vi "Generate GIS Script.vi"(7 "TopLevel in":refnum<class "TopLevel.lvclass">, 8 "error in":errorcluster, 11 "Priming API Data":T1={"Interval (s)"=0.0, "PurgeDuration (s)"=0.0, "Repeats"=0, "PrimingMode"=enum."Pre-Purge", "Head"=enum."1", "Frequency (Hz)"=0, "PrintWeight"=0.1}) -> (0 "error out":errorcluster, 2 "GIS Script":string[](array[string]), 3 "PPScanTrk":T4, 5 "TopLevel out":refnum<class "TopLevel.lvclass">)   [LabVIEW 2022 SP3, in "TopLevel.lvclass"]
uses:
  TopLevel.lvclass
  Typedefs/PrepurgeScanTracking--Cluster.ctl
  Typedefs/PrimingMode APIData.ctl
  Typedefs/PurgeMode--Enum.ctl
  Typedefs/PrinterHeads--Enum.ctl
  IO/Typedefs/ICP1-D0 Channel Names.ctl
  IO/IO.lvclass
panel:
  out "number of replacements":i32
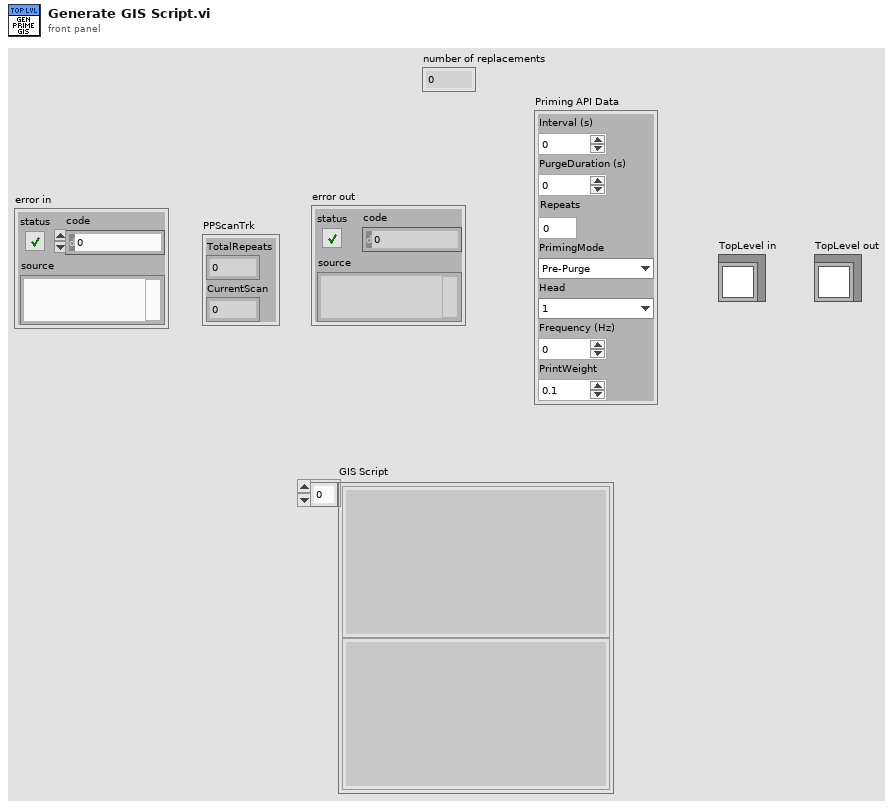
[diagram p1: front panel]
types:
  T1 = typedef "TopLevel.lvclass/PrimingMode APIData.ctl" = cluster{"Interval (s)":dbl, "PurgeDuration (s)":dbl, "Repeats":u8, "PrimingMode":T2, "Head":T3, "Frequency (Hz)":i32, "PrintWeight":dbl}
  T2 = typedef "PurgeMode--Enum.ctl" = enum16{"Pre-Purge", "Purge", "Spit", "Shake"}
  T3 = typedef "PrinterHeads--Enum.ctl" = enum16{"-1", "1", "2", "3", "4", "5", "6"}
  T4 = typedef "PrepurgeScanTracking--Cluster.ctl" = cluster{"TotalRepeats":i32, "CurrentScan":i32}
  T5 = typedef "IO.lvclass/ICP1-D0 Channel Names.ctl" = enum16{"None", "Meniscus Pressure Reg PWR - R1", "Meniscus Pressure Reg PWR - R2", "Meniscus Pressure Reg PWR - R3", "Meniscus Pressure Reg PWR - R4", "Meniscus Pressure Reg PWR - R5", "Meniscus Pressure Reg PWR - R6", "Clear Stage Alarm", "Servo ON", "Purge Valve Open - R1", "Purge Valve Open - R2", "Purge Valve Open - R3", "Purge Valve Open - R4", "Purge Valve Open - R5", "Purge Valve Open - R6"}
  T6 = typedef "DLPConfig)Init_HeadPropertyAttr--Cluster.ctl" = cluster{"HeadNumber":u8, "Material":string, "HeadLocalX":dbl, "HeadLocalY":dbl, "HeadRotationAngle":dbl, "VH2L_Hi":dbl, "VH2R_Hi":dbl, "VH1LA_Hi":dbl, "VH1LB_Hi":dbl, "VH1RA_Hi":dbl, "VH1RB_Hi":dbl, "VH2L_Lo":dbl, "VH2R_Lo":dbl, "VH1LA_Lo":dbl, "VH1LB_Lo":dbl, "VH1RA_Lo":dbl, "VH1RB_Lo":dbl}
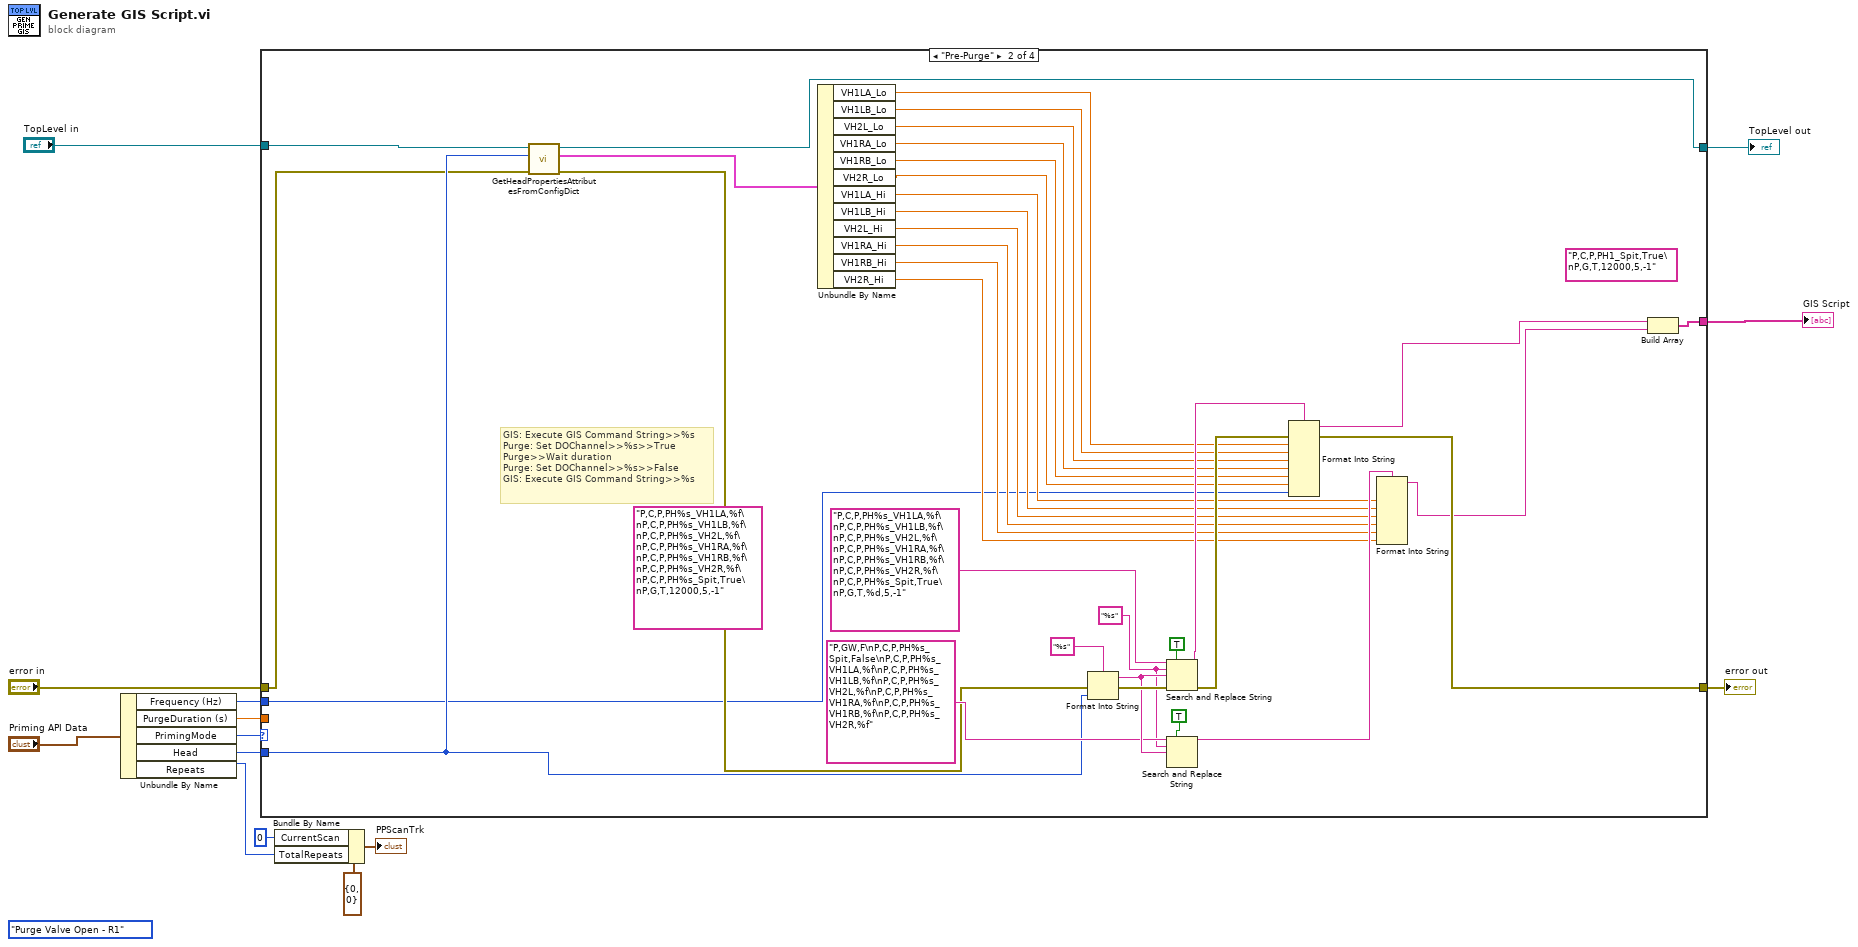
[diagram p0: block diagram]
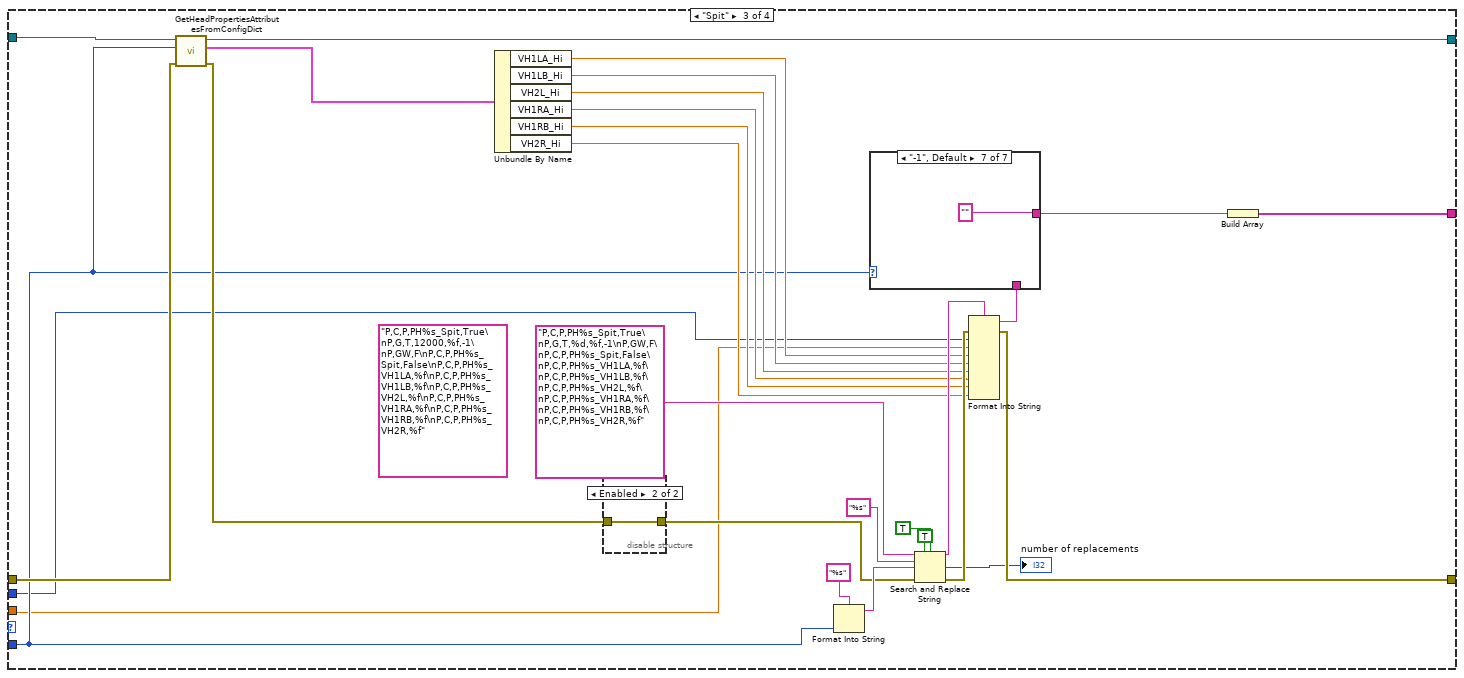
[diagram p3: hidden frame]
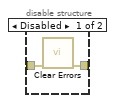
[diagram p4: hidden frame]
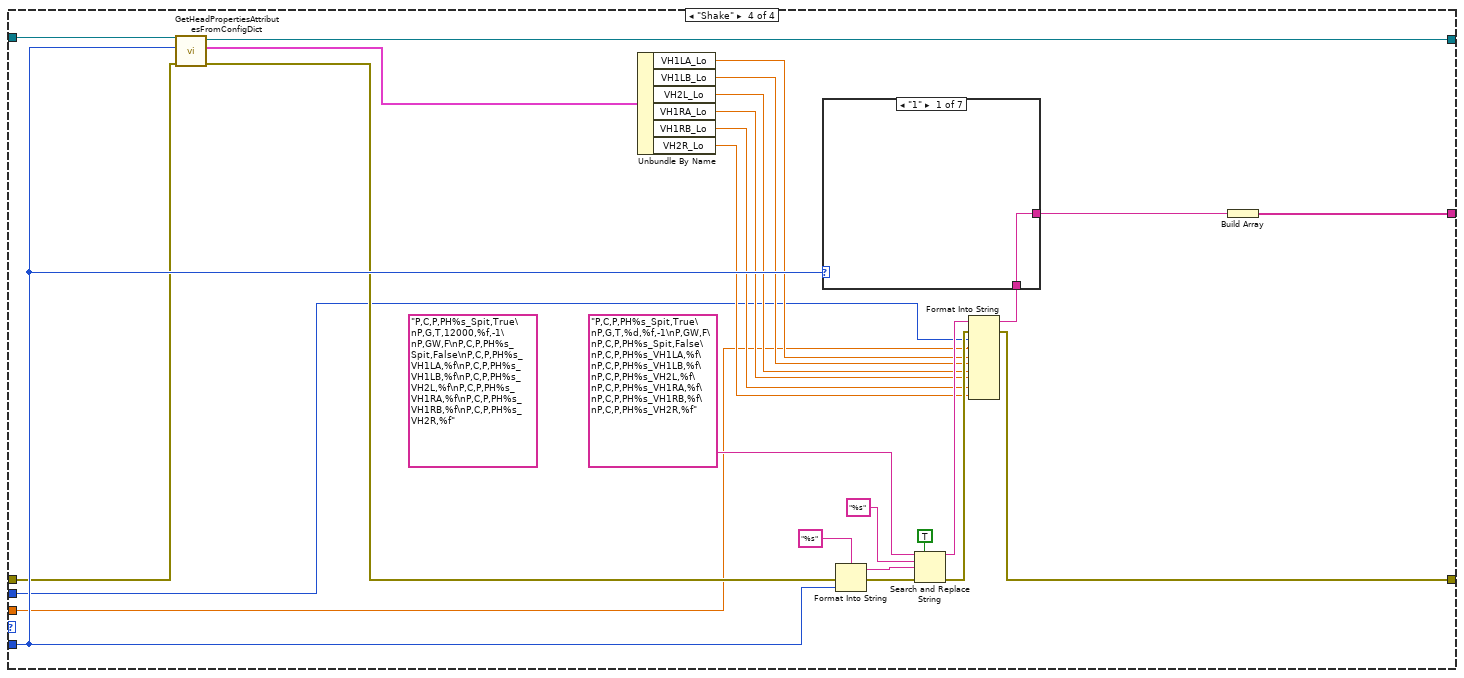
[diagram p11: hidden frame]
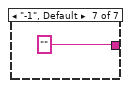
[diagram p17: hidden frame]
diagram:
  (unwired) ICP1-D0_Channel_Names."Purge Valve Open - R1" ("Purge Channel Name")
  n1 = Unbundle By Name("Priming API Data") -> ("Frequency (Hz)"=w1:i32, "PurgeDuration (s)"=w5:dbl, "PrimingMode"=w8:T2, "Head"=w14:T3, "Repeats"=w11:u8)
  n2 = case shown="\"Pre-Purge\"" w8 {
    tunnel: [_ w40 w70 w103] -> w4
    tunnel: w14 -> [_ w34 w57 w100]
    tunnel: "error in" -> [w16 w18 w68 w98]
    tunnel: [w16 w44 w71 w104] -> w6
    tunnel: w5 -> [_ _ w52 w90]
    tunnel: "TopLevel in" -> [w15 w35 w69 w101]
    tunnel: [w15 w20 w67 w97] -> w2
    tunnel: w1 -> [_ w17 w51 w89]
    frame "Purge", Default {
    }
    frame "Pre-Purge" {
      (unwired) "P,C,P,PH%s_VH1LA,%f\nP,C,P,PH%s_VH1LB,%f\nP,C,P,PH%s_VH2L,%f\nP,C,P,PH%s_VH1RA,%f\nP,C,P,PH%s_VH1RB,%f\nP,C,P,PH%s_VH2R,%f\nP,C,P,PH%s_Spit,True\nP,G,T,12000,5,-1" ("format string")
      (unwired) "P,C,P,PH1_Spit,True\nP,G,T,12000,5,-1"
      w37 = "%s" ("search string")
      # "GIS: Execute GIS Command String>>%s\nPurge: Set DOChannel>>%s>>True\nPurge>>Wait duration\nPurge: Set DOChannel>>%s>>False\nGIS: Execute GIS Command String>>%s"
      n3 = call "GetHeadPropertiesAttributesFromConfigDict.vi"("error in (no error)"=w18, "Head"=w34, "TopLevel in"=w35) -> ("error out"=w19:errorcluster, "#attributes"=w33:T6, "TopLevel out"=w20:refnum<class "TopLevel.lvclass">)  [unwired: 5 in, 1 out]
      n4 = Unbundle By Name(w33) -> ("VH1LA_Lo"=w32:dbl, "VH1LB_Lo"=w31:dbl, "VH2L_Lo"=w30:dbl, "VH1RA_Lo"=w29:dbl, "VH1RB_Lo"=w28:dbl, "VH2R_Lo"=w27:dbl, "VH1LA_Hi"=w26:dbl, "VH1LB_Hi"=w25:dbl, "VH2L_Hi"=w24:dbl, "VH1RA_Hi"=w23:dbl, "VH1RB_Hi"=w22:dbl, "VH2R_Hi"=w21:dbl)
      n5 = Format Into String(format string="%s", error in=w19, w34) -> (resulting string=w42:string, error out=w47:errorcluster)  [unwired: 1 in]
      n6 = Search and Replace String(replace all?=TRUE ("replace all? (F)"), input string="P,C,P,PH%s_VH1LA,%f\nP,C,P,PH%s_VH1LB,%f\nP,C,P,PH%s_VH2L,%f\nP,C,P,PH%s_VH1RA,%f\nP,C,P,PH%s_VH1RB,%f\nP,C,P,PH%s_VH2R,%f\nP,C,P,PH%s_Spit,True\nP,G,T,%d,5,-1" ("format string"), search string=w37, replace string=w42, error in=w47) -> (result string=w46:string, error out=w45:errorcluster)  [unwired: 3 in, 2 out]
      n7 = Search and Replace String(replace all?=TRUE ("replace all? (F)"), input string="P,GW,F\nP,C,P,PH%s_Spit,False\nP,C,P,PH%s_VH1LA,%f\nP,C,P,PH%s_VH1LB,%f\nP,C,P,PH%s_VH2L,%f\nP,C,P,PH%s_VH1RA,%f\nP,C,P,PH%s_VH1RB,%f\nP,C,P,PH%s_VH2R,%f" ("format string"), search string=w37, replace string=w42) -> (result string=w41:string)  [unwired: 4 in, 3 out]
      n8 = Format Into String(format string=w46, error in=w45, w32, w31, w30, w29, w28, w27, w17) -> (resulting string=w36:string, error out=w44:errorcluster)  [unwired: 1 in]
      n9 = Format Into String(format string=w41, w26, w25, w24, w23, w22, w21) -> (resulting string=w39:string)  [unwired: 2 in, 1 out]
      n10 = Build Array(w36, w39) -> (w40:string[])
    }
    frame "Spit" {
      (unwired) "P,C,P,PH%s_Spit,True\nP,G,T,12000,%f,-1\nP,GW,F\nP,C,P,PH%s_Spit,False\nP,C,P,PH%s_VH1LA,%f\nP,C,P,PH%s_VH1LB,%f\nP,C,P,PH%s_VH2L,%f\nP,C,P,PH%s_VH1RA,%f\nP,C,P,PH%s_VH1RB,%f\nP,C,P,PH%s_VH2R,%f" ("format string")
      n11 = call "GetHeadPropertiesAttributesFromConfigDict.vi"("error in (no error)"=w68, "Head"=w57, "TopLevel in"=w69) -> ("error out"=w58:errorcluster, "#attributes"=w66:T6, "TopLevel out"=w67:refnum<class "TopLevel.lvclass">)  [unwired: 5 in, 1 out]
      n12 = Unbundle By Name(w66) -> ("VH1LA_Hi"=w65:dbl, "VH1LB_Hi"=w64:dbl, "VH2L_Hi"=w63:dbl, "VH1RA_Hi"=w62:dbl, "VH1RB_Hi"=w61:dbl, "VH2R_Hi"=w60:dbl)
      n13 = disable-structure shown="Enabled" {
        disable-tunnel: w58 -> [w80 w81]
        disable-tunnel: [w79 w81] -> w53
        frame Disabled {
          n14 = call <vilib>:"Clear Errors.vi"("error in (no error)"=w80) -> ("error out"=w79:errorcluster)  [unwired: 5 in, 1 out]
        }
        frame Enabled {
        }
      }
      n15 = Format Into String(format string="%s", w57) -> (resulting string=w56:string)  [unwired: 2 in, 1 out]
      n16 = Search and Replace String(replace all?=TRUE ("replace all? (F)"), case sensitive?=TRUE ("ignore case? (F)"), input string="P,C,P,PH%s_Spit,True\nP,G,T,%d,%f,-1\nP,GW,F\nP,C,P,PH%s_Spit,False\nP,C,P,PH%s_VH1LA,%f\nP,C,P,PH%s_VH1LB,%f\nP,C,P,PH%s_VH2L,%f\nP,C,P,PH%s_VH1RA,%f\nP,C,P,PH%s_VH1RB,%f\nP,C,P,PH%s_VH2R,%f" ("format string"), search string="%s", replace string=w56, error in=w53) -> (result string=w74:string, number of replacements=→"number of replacements":i32, error out=w72:errorcluster)  [unwired: 2 in, 1 out]
      n17 = Format Into String(format string=w74, error in=w72, w51, w52, w65, w64, w63, w62, w61, w60) -> (resulting string=w73:string, error out=w71:errorcluster)  [unwired: 1 in]
      n18 = case shown="\"-1\", Default" w57 {
        tunnel: w73 -> [w82 w83 w84 w85 w86 w87 _]
        tunnel: [w82 w83 w84 w85 w86 w87 "" ("result string")] -> w75
        frame "1" {
        }
        frame "2" {
        }
        frame "3" {
        }
        frame "4" {
        }
        frame "5" {
        }
        frame "6" {
        }
        frame "-1", Default {
        }
      }
      n19 = Build Array(w75) -> (w70:string[])
    }
    frame "Shake" {
      (unwired) "P,C,P,PH%s_Spit,True\nP,G,T,12000,%f,-1\nP,GW,F\nP,C,P,PH%s_Spit,False\nP,C,P,PH%s_VH1LA,%f\nP,C,P,PH%s_VH1LB,%f\nP,C,P,PH%s_VH2L,%f\nP,C,P,PH%s_VH1RA,%f\nP,C,P,PH%s_VH1RB,%f\nP,C,P,PH%s_VH2R,%f" ("format string")
      n20 = call "GetHeadPropertiesAttributesFromConfigDict.vi"("error in (no error)"=w98, "Head"=w100, "TopLevel in"=w101) -> ("error out"=w99:errorcluster, "#attributes"=w102:T6, "TopLevel out"=w97:refnum<class "TopLevel.lvclass">)  [unwired: 5 in, 1 out]
      n21 = Unbundle By Name(w102) -> ("VH1LA_Lo"=w96:dbl, "VH1LB_Lo"=w95:dbl, "VH2L_Lo"=w94:dbl, "VH1RA_Lo"=w93:dbl, "VH1RB_Lo"=w92:dbl, "VH2R_Lo"=w91:dbl)
      n22 = Format Into String(format string="%s", error in=w99, w100) -> (resulting string=w111:string, error out=w109:errorcluster)  [unwired: 1 in]
      n23 = Search and Replace String(replace all?=TRUE ("replace all? (F)"), input string="P,C,P,PH%s_Spit,True\nP,G,T,%d,%f,-1\nP,GW,F\nP,C,P,PH%s_Spit,False\nP,C,P,PH%s_VH1LA,%f\nP,C,P,PH%s_VH1LB,%f\nP,C,P,PH%s_VH2L,%f\nP,C,P,PH%s_VH1RA,%f\nP,C,P,PH%s_VH1RB,%f\nP,C,P,PH%s_VH2R,%f" ("format string"), search string="%s", replace string=w111, error in=w109) -> (result string=w107:string, error out=w105:errorcluster)  [unwired: 3 in, 2 out]
      n24 = Format Into String(format string=w107, error in=w105, w89, w90, w96, w95, w94, w93, w92, w91) -> (resulting string=w106:string, error out=w104:errorcluster)  [unwired: 1 in]
      n25 = case shown="\"1\"" w100 {
        tunnel: w106 -> [w115 w116 w117 w118 w119 w120 _]
        tunnel: [w115 w116 w117 w118 w119 w120 "" ("result string")] -> w108
        frame "1" {
        }
        frame "2" {
        }
        frame "3" {
        }
        frame "4" {
        }
        frame "5" {
        }
        frame "6" {
        }
        frame "-1", Default {
        }
      }
      n26 = Build Array(w108) -> (w103:string[])
    }
  }
  "error out" <- w6
  "GIS Script" <- w4
  "TopLevel out" <- w2
  n27 = Bundle By Name(cluster=T4 {"TotalRepeats"=0, "CurrentScan"=0} ("PPScanTrk"), "CurrentScan"=0 ("PPScanTrk.CurrentScan"), "TotalRepeats"=w11) -> (→"PPScanTrk":T4)
